vi "Calculate C2V.vi"(9 "Tcal_Chamber":dbl, 10 "CO2":dbl caption="Calibration Gas Concentration" format="%_6g", 11 "Calibration Coefficients":T1={"CalFile Used"=path "", "TYPE"="", "DATE"="", "Humidity"=0.0, "Chamber Temp"=0.0, "CO2_calgas"=nan, "V_(RA,5mA)"=nan, "V_(RA,15mA)"=nan, "mI"=nan, "V_0d_ImA (actual)"=nan, "V_6d_ImA (actual)"=nan, "I_span"=nan, "DAC"=0, "A"=nan, "B"=nan, "C"=nan, "D"=nan, "V6d"=nan, "A'"=0.0, "B'"=0.0, "C'"=0.0, "D'"=0.0, "V0d"=0.0, "CalDate"="", "CalTime"="", "duration"=0.0, "Detector Channel"="", "a2"=nan, "a3"=nan, "a4"=nan, "a5"=nan, "b2"=nan, "c2"=nan, "b3"=nan, "c3"=nan, "b4"=nan, "c4"=nan, "b5"=nan, "c5"=nan, "a7"=nan, "a8"=nan, "a9"=nan, "a10"=nan, "b7"=nan, "b8"=nan, "b9"=nan, "b10"=nan, "c7"=nan, "c8"=nan, "c9"=nan, "c10"=nan, "cal_offs_adj"=0.0, "cal_gain_adj"=1.0, "C6d"=nan, "C0d"=0.0, "Cal_currernt"=nan, "C2V"=0, "V2C"=0, "Zero Date"="", "Zero Time"="", "Number of Zeroes"=0, "V_(()d, average)"=nan, "V_offs "=0.0, "G_adj"=1.0, "Pump Flow Rate"=0, "Zero Required? "=FALSE, "Calibrate Required?"=FALSE, "cal_utc"=0.0, "zero_utc"=0.0, "Elapsed Time"=0.0, "PCB"="", "m0"=0.0, "b0"=0.0} {"Elapsed Time" format="%<%H:%M:%S>t"; "Pump Flow Rate" format="%0d"; "Number of Zeroes" format="%0d"; "V2C" format="%0d"; "C2V" format="%0d"; "duration" format="%<%H:%M:%S>t"; "DAC" format="%03x"; "mI" format="%.3g"; "V_(RA,15mA)" format="%0.4f"; "V_(RA,5mA)" format="%0.4f"; "Chamber Temp" format="%.1f"; "Humidity" format="%.1f"}) -> (3 "Calibration Coefficients Out":T1={"CalFile Used"=path "", "TYPE"="", "DATE"="", "Humidity"=0.0, "Chamber Temp"=0.0, "CO2_calgas"=nan, "V_(RA,5mA)"=nan, "V_(RA,15mA)"=nan, "mI"=nan, "V_0d_ImA (actual)"=nan, "V_6d_ImA (actual)"=nan, "I_span"=nan, "DAC"=0, "A"=nan, "B"=nan, "C"=nan, "D"=nan, "V6d"=nan, "A'"=0.0, "B'"=0.0, "C'"=0.0, "D'"=0.0, "V0d"=0.0, "CalDate"="", "CalTime"="", "duration"=0.0, "Detector Channel"="", "a2"=nan, "a3"=nan, "a4"=nan, "a5"=nan, "b2"=nan, "c2"=nan, "b3"=nan, "c3"=nan, "b4"=nan, "c4"=nan, "b5"=nan, "c5"=nan, "a7"=nan, "a8"=nan, "a9"=nan, "a10"=nan, "b7"=nan, "b8"=nan, "b9"=nan, "b10"=nan, "c7"=nan, "c8"=nan, "c9"=nan, "c10"=nan, "cal_offs_adj"=0.0, "cal_gain_adj"=1.0, "C6d"=nan, "C0d"=0.0, "Cal_currernt"=nan, "C2V"=0, "V2C"=0, "Zero Date"="", "Zero Time"="", "Number of Zeroes"=0, "V_(()d, average)"=nan, "V_offs "=0.0, "G_adj"=1.0, "Pump Flow Rate"=0, "Zero Required? "=FALSE, "Calibrate Required?"=FALSE, "cal_utc"=0.0, "zero_utc"=0.0, "Elapsed Time"=0.0, "PCB"="", "m0"=0.0, "b0"=0.0} {"Elapsed Time" format="%<%H:%M:%S>t"; "Pump Flow Rate" format="%0d"; "Number of Zeroes" format="%0d"; "V2C" format="%0d"; "C2V" format="%0d"; "duration" format="%<%H:%M:%S>t"; "DAC" format="%03x"; "mI" format="%.3g"; "V_(RA,15mA)" format="%0.4f"; "V_(RA,5mA)" format="%0.4f"; "Chamber Temp" format="%.1f"; "Humidity" format="%.1f"})   [LabVIEW 2016]
uses:
  Controls/Calibration Coefficients.ctl
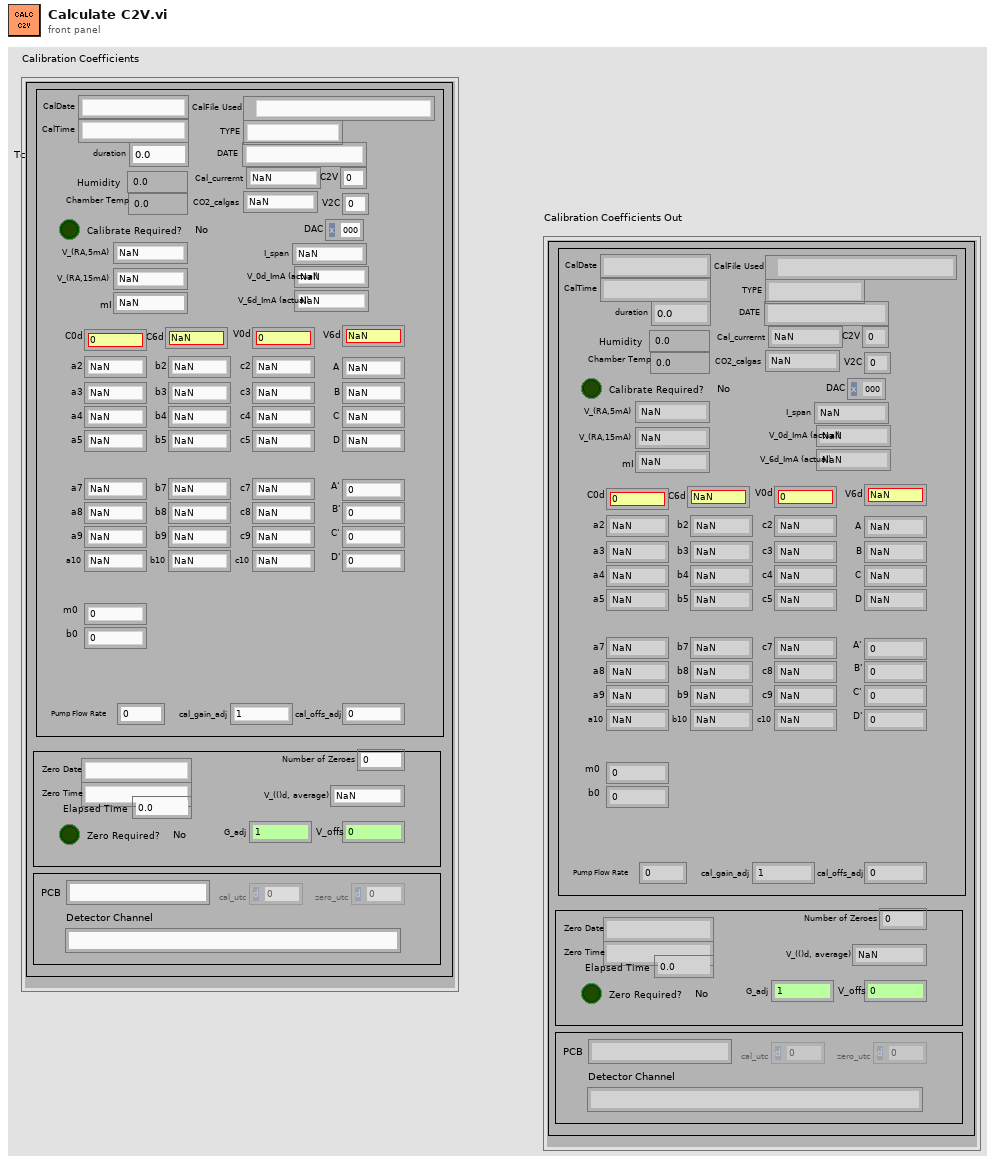
[diagram p1: front panel]
types:
  T1 = typedef "Calibration Coefficients.ctl" = cluster{"CalFile Used":path, "TYPE":string, "DATE":string, "Humidity":sgl, "Chamber Temp":dbl, "CO2_calgas":dbl, "V_(RA,5mA)":dbl, "V_(RA,15mA)":dbl, "mI":dbl, "V_0d_ImA (actual)":dbl, "V_6d_ImA (actual)":dbl, "I_span":dbl, "DAC":u16, "A":dbl, "B":dbl, "C":dbl, "D":dbl, "V6d":dbl, "A'":dbl, "B'":dbl, "C'":dbl, "D'":dbl, "V0d":dbl, "CalDate":string, "CalTime":string, "duration":dbl, "Detector Channel":string, "a2":dbl, "a3":dbl, "a4":dbl, "a5":dbl, "b2":dbl, "c2":dbl, "b3":dbl, "c3":dbl, "b4":dbl, "c4":dbl, "b5":dbl, "c5":dbl, "a7":dbl, "a8":dbl, "a9":dbl, "a10":dbl, "b7":dbl, "b8":dbl, "b9":dbl, "b10":dbl, "c7":dbl, "c8":dbl, "c9":dbl, "c10":dbl, "cal_offs_adj":dbl, "cal_gain_adj":dbl, "C6d":dbl, "C0d":dbl, "Cal_currernt":dbl, "C2V":u16, "V2C":u16, "Zero Date":string, "Zero Time":string, "Number of Zeroes":u16, "V_(()d, average)":dbl, "V_offs ":dbl, "G_adj":dbl, "Pump Flow Rate":u16, "Zero Required? ":bool, "Calibrate Required?":bool, "cal_utc":dbl, "zero_utc":dbl, "Elapsed Time":dbl, "PCB":string, "m0":dbl, "b0":dbl}
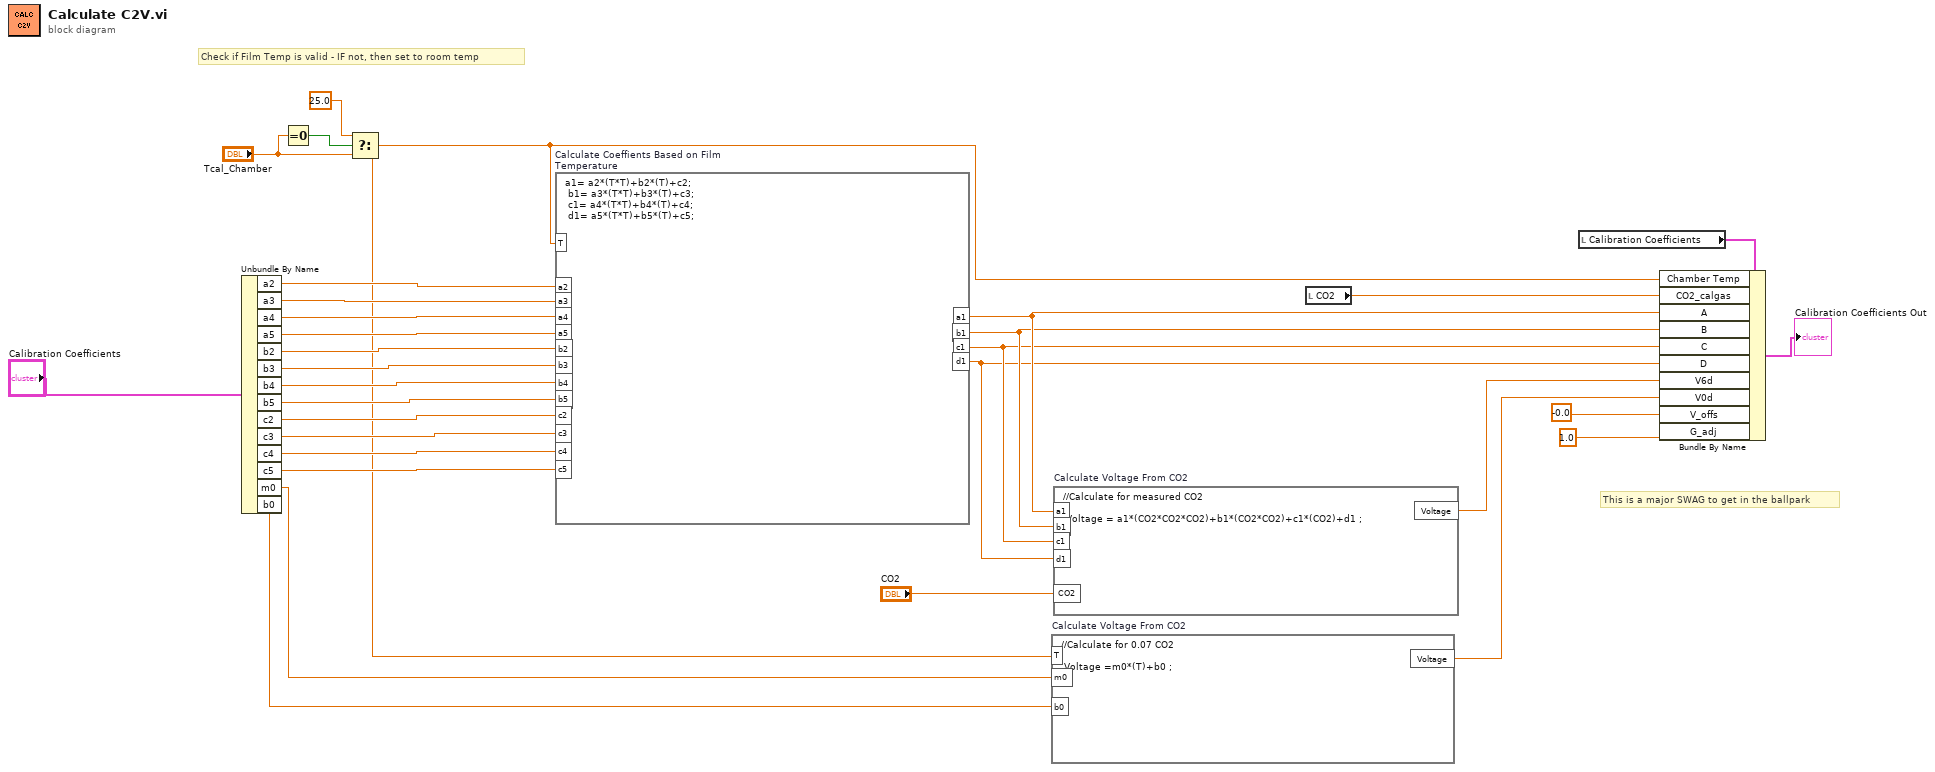
[diagram p0: block diagram]
diagram:
  # "This is a major SWAG to get in the ballpark"
  # "Check if Film Temp is valid - IF not, then set to room temp"
  n1 = Unbundle By Name("Calibration Coefficients") -> ("a2"=w31:dbl, "a3"=w30:dbl, "a4"=w29:dbl, "a5"=w28:dbl, "b2"=w27:dbl, "b3"=w26:dbl, "b4"=w25:dbl, "b5"=w24:dbl, "c2"=w23:dbl, "c3"=w22:dbl, "c4"=w21:dbl, "c5"=w20:dbl, "m0"=w2:dbl, "b0"=w1:dbl)
  n2 = Equal To 0?(x="Tcal_Chamber") -> (x = 0?=w10:bool)
  n3 = Select(t=25.0, s=w10, f="Tcal_Chamber") -> (s? t:f=w3:dbl)
  n4 = formula code="a1=\ta2*(T*T)+b2*(T)+c2;\n\tb1=\ta3*(T*T)+b3*(T)+c3;\n\tc1=\ta4*(T*T)+b4*(T)+c4;\n\td1=\ta5*(T*T)+b5*(T)+c5;" "Calculate Coeffients Based on Film Temperature"("T"=w3, "a2"=w31, "a3"=w30, "a4"=w29, "a5"=w28, "b2"=w27, "b3"=w26, "b4"=w25, "b5"=w24, "c2"=w23, "c3"=w22, "c4"=w21, "c5"=w20) -> ("a1"=w17:dbl, "b1"=w16:dbl, "c1"=w15:dbl, "d1"=w14:dbl)
  n5 = formula code="//Calculate for 0.07 CO2\n\n\tVoltage =m0*(T)+b0\t;" "Calculate Voltage From CO2"("T"=w3, "m0"=w2, "b0"=w1) -> ("Voltage"=w7:dbl)
  n6 = formula code="//Calculate for measured CO2\n\n\tVoltage =\ta1*(CO2*CO2*CO2)+b1*(CO2*CO2)+c1*(CO2)+d1\t;" "Calculate Voltage From CO2"("a1"=w17, "b1"=w16, "c1"=w15, "d1"=w14, "CO2"="CO2") -> ("Voltage"=w8:dbl)
  n7 = local read "CO2"() -> (w18:dbl)
  n8 = local read "Calibration Coefficients"() -> (w19:T1)
  n9 = Bundle By Name(cluster=w19, "Chamber Temp"=w3, "CO2_calgas"=w18, "A"=w17, "B"=w16, "C"=w15, "D"=w14, "V6d"=w8, "V0d"=w7, "V_offs"=-0.0, "G_adj"=1.0) -> (→"Calibration Coefficients Out":T1)
